vi "GetErdName.vi"(0 "session in":refnum<k35>, 7 "Input Erd":string, 11 "error in":errorcluster) -> (4 "session out":refnum<k35>, 8 "Erd Name":string, 15 "error out":errorcluster)   [LabVIEW 2021]
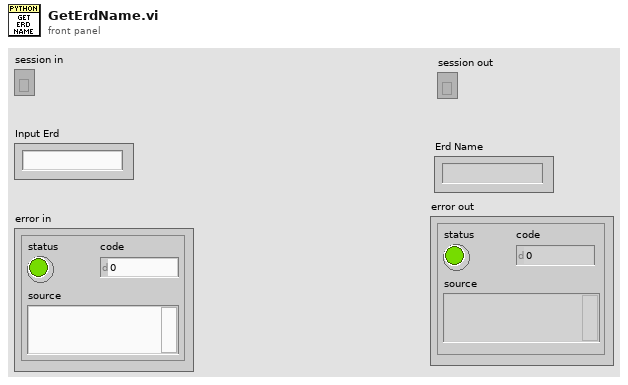
[diagram p1: front panel]
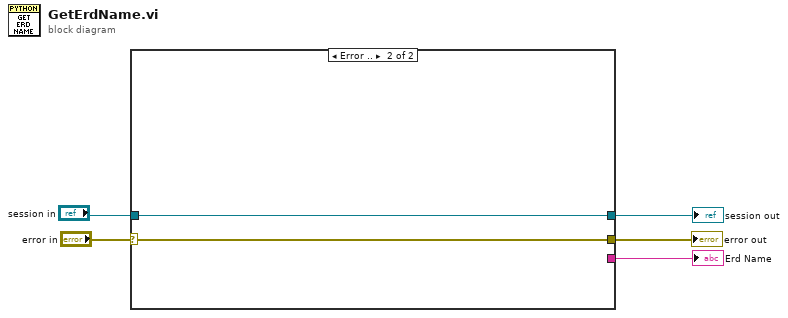
[diagram p0: block diagram]
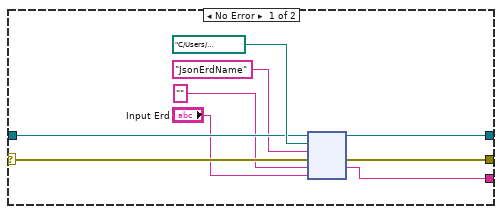
[diagram p2: hidden frame]
diagram:
  n1 = case shown="Error .." "error in" {
    selector: "error in" -> [w13 w16]
    tunnel: [w11 w16] -> w5
    tunnel: "session in" -> [w12 w15]
    tunnel: [w10 w15] -> w2
    tunnel: [w6 _] -> w1
    frame No Error {
      n2 = node(w12, path "C:/Users/LNLMEXID/Desktop/Python/AT-LabView-Python/src/Main.py" ("module path"), "JsonErdName" ("function name"), w13, "" ("function name"), "Input Erd") -> (w10:refnum<k35>, w11:errorcluster, w6:string)  [unwired: 1 in, 2 out]
    }
    frame Error {
    }
  }
  "error out" <- w5
  "session out" <- w2
  "Erd Name" <- w1
